vi "8.8.3_b.vi"() -> ()   [LabVIEW 2018]
panel:
  in  "b정지":bool
  out "b":dbl(graph)
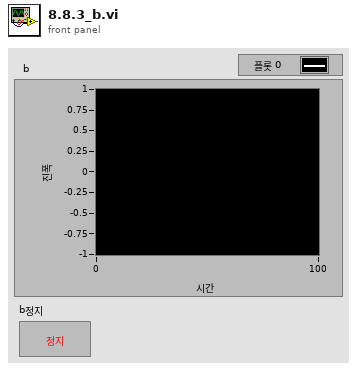
[diagram p1: front panel]
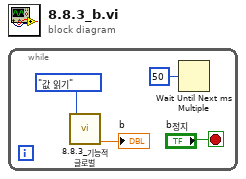
[diagram p0: block diagram]
diagram:
  n1 = while {
    stop <- "b정지" stop-if-true
    n2 = call "8.8.3_기능적 글로벌.vi"("명령"=enum16{"값 쓰기", "값 읽기"}."값 읽기") -> ("출력"=→"b":dbl)  [unwired: 2 in]
    n3 = Wait Until Next ms Multiple(millisecond multiple=u32 50 ("ms 배수")) -> ()  [unwired: 1 out]
  }
